vi "Private Test.vi"() -> ()   [LabVIEW 2016, in "Assert API Components.lvlib" / "Log Assert Core.lvlib" / "Abort Application Unit Test.lvclass"]
uses:
  Abort Application Unit Test.lvclass
panel:
  out "Numeric":i32
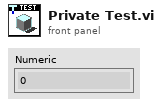
[diagram p1: front panel]
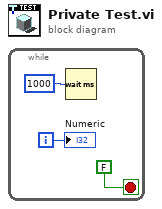
[diagram p0: block diagram]
diagram:
  n1 = while {
    i -> [w1]
    stop <- FALSE stop-if-true
    n2 = Wait (ms)(milliseconds to wait=u32 1000) -> ()  [unwired: 1 out]
    "Numeric" <- w1
  }
